vi "WFComposeD.vi"(8 "error in (no error)":errorcluster, 10 "WFRepetitions":T1={"Del (s)"=0.0, "Int (s)"=0.0, "N"=1} {"Int (s)" min=0.0 format="%#_4g"; "Del (s)" min=0.0 format="%#_4f"}, 11 "Waveform In":digitalwaveform(waveform)={"t0"=timestamp(0 s since 1904-01-01), "dt"=1.0, "Y"={"transitions"=[], "data"=[[0, 0, 0, 1], [0, 1, 0, 0]]}}) -> (0 "error out":errorcluster, 3 "Waveform Out":digitalwaveform(waveform)={"t0"=timestamp(0 s since 1904-01-01), "dt"=1.0, "Y"={"transitions"=[], "data"=[[0, 0, 0, 1], [0, 1, 0, 0]]}})   [LabVIEW 2013]
uses:
  WFRepetitions.ctl
  WFComposeCanD.vi
  WFGetDtFsD.vi
  <vilib>/Waveform/DWDTOps.llb/DWDT Digital Size.vi
  <vilib>/Waveform/DWDTOps.llb/DWDT Boolean Array to Digital.vi
  WFAppend2D.vi
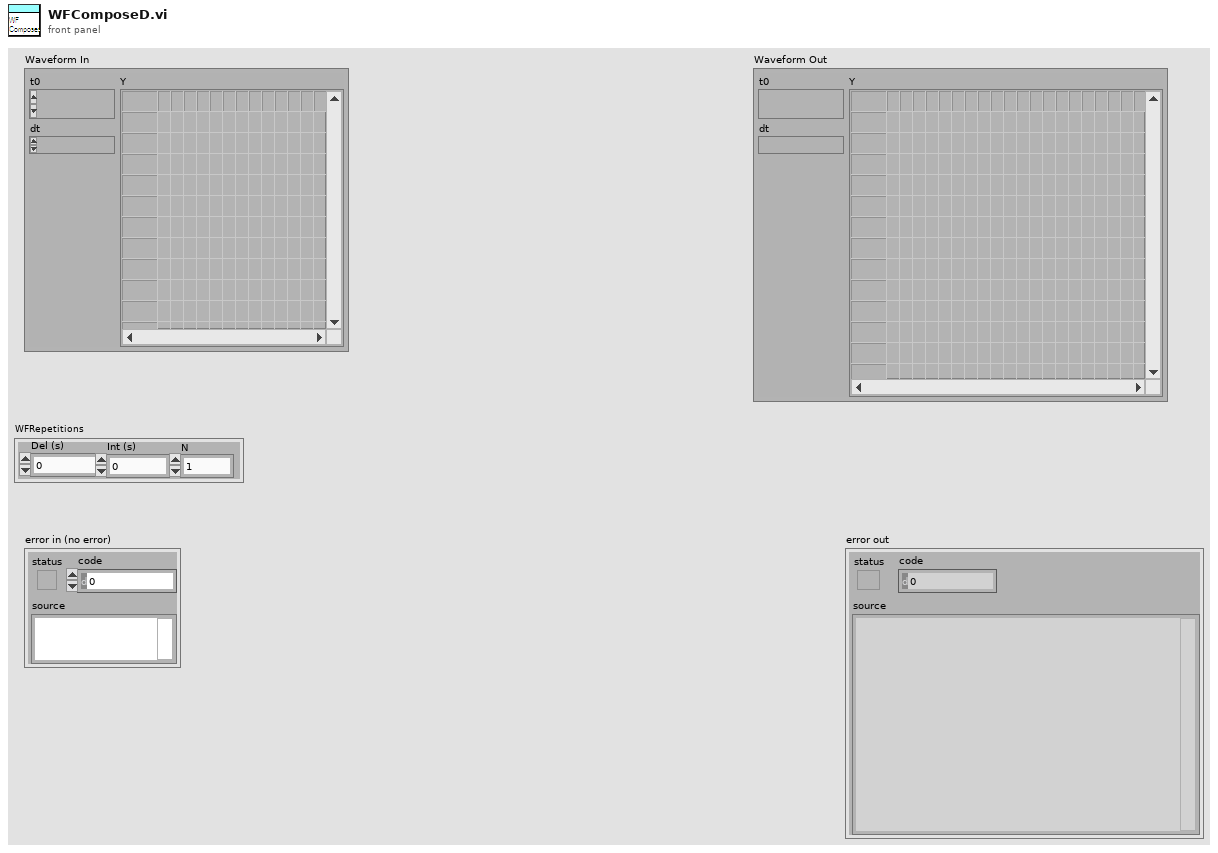
[diagram p1: front panel]
types:
  T1 = typedef "WFRepetitions.ctl" = cluster{"Del (s)":dbl, "Int (s)":dbl, "N":i32}
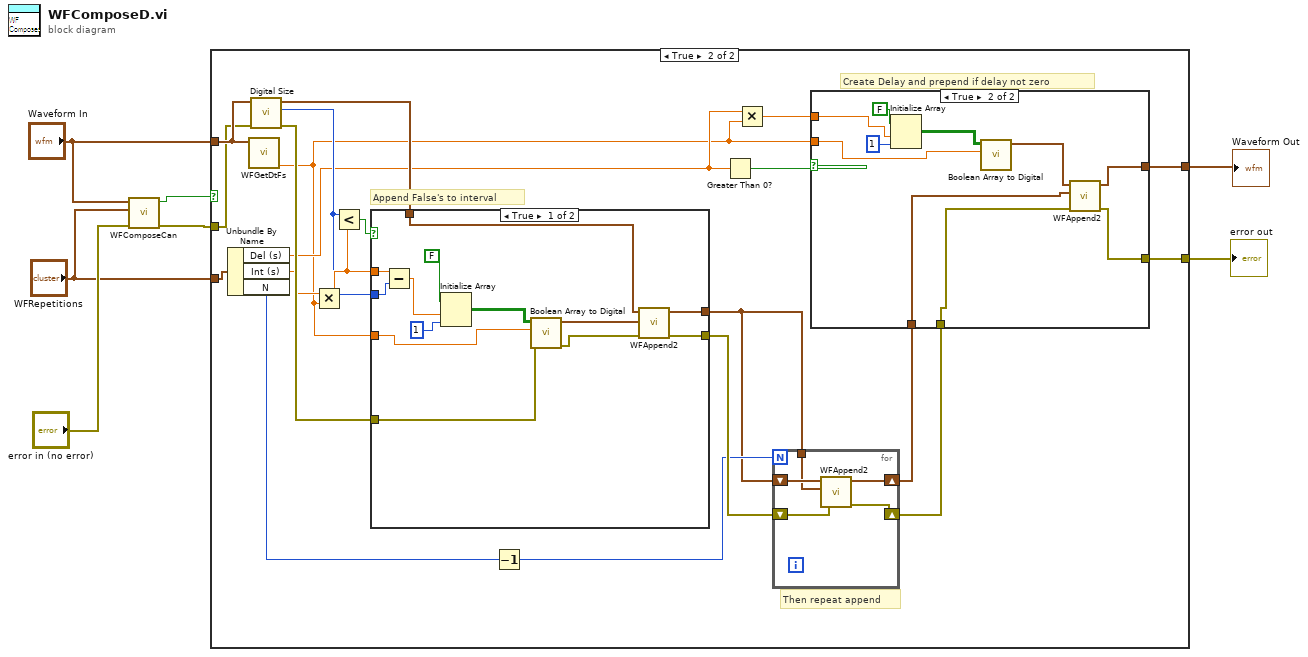
[diagram p0: block diagram]
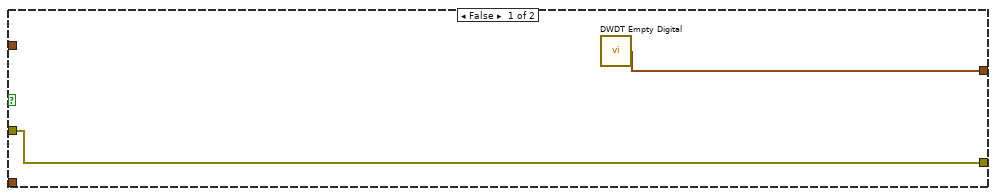
[diagram p2: hidden frame]
diagram:
  n1 = call-poly "WFComposeCan.vi"("error in (no error)"="error in (no error)", "Cluster"="WFRepetitions", "Waveform In"="Waveform In") -> ("error out"=w5:errorcluster, "ComposeCan"=w7:bool)  [unwired: 7 in]
  n2 = case shown="True" w7 {
    tunnel: [w8 w18] -> w1
    tunnel: w5 -> [w9 w24]
    tunnel: [w9 w16] -> w4
    tunnel: "Waveform In" -> [_ w27]
    tunnel: "WFRepetitions" -> [_ w28]
    frame False {
      n3 = call <vilib>:"DWDT Empty Digital.vi"() -> ("digital waveform out"=w8:digitalwaveform)  [unwired: 5 in]
    }
    frame True {
      # "Then repeat append"
      # "Create Delay and prepend if delay not zero"
      # "Append False's to interval"
      n4 = Unbundle By Name(w28) -> ("Del (s)"=w12:dbl, "Int (s)"=w15:dbl, "N"=w22:i32)
      n5 = call-poly "WFGetDtFs.vi"("Waveform"=w27) -> ("Fs (Hz)"=w10:dbl)  [unwired: 9 in, 1 out]
      n6 = call-poly <vilib>:"Digital Size.vi"("error in (no error)"=w24, "digital waveform in"=w27) -> ("error out"=w23:errorcluster, "number of samples"=w13:i32, "digital waveform out"=w25:digitalwaveform)  [unwired: 6 in, 1 out]
      n7 = Multiply(x=w15, y=w10) -> (x*y=w14:dbl)
      n8 = Less?(x=w13, y=w14) -> (x < y?=w26:bool)
      n9 = case shown="True" w26 {
        tunnel: [w46 w50] -> w29
        tunnel: [w45 w49] -> w20
        tunnel: w25 -> [w39 w49]
        tunnel: w14 -> [w38 _]
        tunnel: w23 -> [w42 w50]
        tunnel: w13 -> [w37 _]
        tunnel: w10 -> [w36 _]
        frame True {
          n10 = Subtract(x=w38, y=w37) -> (x-y=w47:dbl)
          n11 = Initialize Array(FALSE, w47, 1 ("dimension size")) -> (w43:bool[][])
          n12 = call-poly <vilib>:"Boolean Array to Digital.vi"("error in (no error)"=w42, "sample rate"=w36, "boolean array"=w43) -> ("error out"=w41:errorcluster, "digital waveform"=w40:digitalwaveform)  [unwired: 7 in]
          n13 = call-poly "WFAppend2.vi"("error in (no error)"=w41, "Waveform In 2"=w40, "Waveform In"=w39) -> ("error out"=w46:errorcluster, "Waveform Out"=w45:digitalwaveform)  [unwired: 3 in]
        }
        frame False {
        }
      }
      n14 = Decrement(x=w22) -> (x-1=w21:i32)
      n15 = Greater Than 0?(x=w12) -> (x > 0?=w30:bool)
      n16 = Multiply(x=w12, y=w10) -> (x*y=w11:dbl)
      n17 = for {
        N: w21 -> [_]
        shift-right: [w34] -> w19
        shift-left: w20 -> [w35]
        shift-right: [w32] -> w17
        shift-left: w29 -> [w33]
        tunnel: w20 -> [w31]
        n18 = call-poly "WFAppend2.vi"("error in (no error)"=w33, "Waveform In 2"=w31, "Waveform In"=w35) -> ("error out"=w32:errorcluster, "Waveform Out"=w34:digitalwaveform)  [unwired: 3 in]
      }
      n19 = case shown="True" w30 {
        tunnel: w10 -> [_ w57]
        tunnel: w19 -> [w52 w55]
        tunnel: [w52 w54] -> w18
        tunnel: w17 -> [w51 w62]
        tunnel: [w51 w61] -> w16
        tunnel: w11 -> [_ w53]
        frame False {
        }
        frame True {
          n20 = Initialize Array(FALSE, w53, 1 ("dimension size")) -> (w58:bool[][])
          n21 = call-poly <vilib>:"Boolean Array to Digital.vi"("sample rate"=w57, "boolean array"=w58) -> ("digital waveform"=w56:digitalwaveform)  [unwired: 8 in, 1 out]
          n22 = call-poly "WFAppend2.vi"("error in (no error)"=w62, "Waveform In 2"=w55, "Waveform In"=w56) -> ("error out"=w61:errorcluster, "Waveform Out"=w54:digitalwaveform)  [unwired: 3 in]
        }
      }
    }
  }
  "error out" <- w4
  "Waveform Out" <- w1
